vi "Rename BaseNodeType if not Empty.vi"(8 "error in":errorcluster, 10 "name":string, 11 "BaseNodeType in":refnum<k39>) -> (0 "error out":errorcluster, 3 "BaseNodeType out":refnum<k39>)   [LabVIEW 2020, in "Custom Device Serialization.lvlib"]
uses:
  Custom Device Serialization.lvlib
  C:/NetCoreDLL/NationalInstruments.VeriStand.SystemStorage.dll
  NetCoreDLL/NationalInstruments.VeriStand.SystemStorage.dll
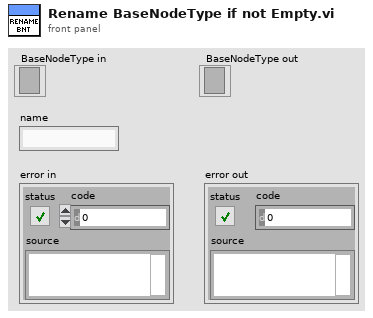
[diagram p1: front panel]
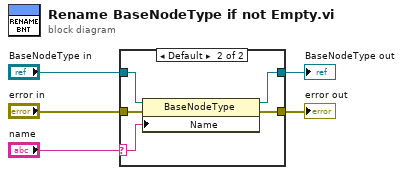
[diagram p0: block diagram]
diagram:
  n1 = case shown="Default" "name" {
    selector: "name" -> [_ w8]
    tunnel: "error in" -> [w6 w12]
    tunnel: [w6 w11] -> w2
    tunnel: "BaseNodeType in" -> [w7 w10]
    tunnel: [w7 w9] -> w4
    frame "" {
    }
    frame Default {
      n2 = property class="BaseNodeType"(reference=w10, error in=w12, "Name"=w8) -> (reference out=w9:refnum<k39>, error out=w11:errorcluster)
    }
  }
  "BaseNodeType out" <- w4
  "error out" <- w2
